vi "FTW-Test-JSON-InvalidPath.vi"() -> (0 "Test Result":errorcluster {"code" format="%.0x"})   [LabVIEW 2015]
uses:
  src/json/FTW-JSON-Type.ctl
  src/json/core/FTW-JSON-Core-Type.ctl
  lib/FTW-KernelFilepath.vi
  src/json/core/FTW-JSON-Core-LibraryReturnValue.vi
  src/error/FTW-ERR-ThrowInvalidReferenceError.vi
  src/json/core/FTW-JSON-Core-ElementType.vi
  codegen/xnode/FTW-JSON-Fetch.xnode
  src/core/type/FTW-Type-JSON.ctl
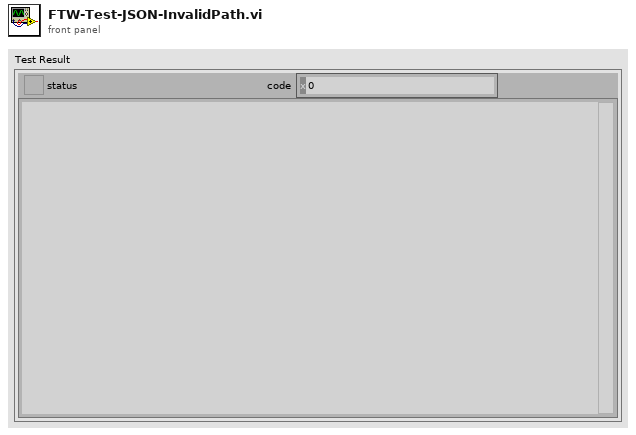
[diagram p1: front panel]
types:
  T1 = typedef "FTW-JSON-Type.ctl" = enum8{"Not Found", "Object", "Array", "String", "Number", "Boolean", "null"}
  T2 = cluster{"Path":string, "ExpectedValue":i32, "ExpectedType":T1, "ExpectedError":bool}[]
  T3 = typedef "FTW-Type-JSON.ctl" = refnum<data-value>
  T4 = typedef "FTW-JSON-Core-Type.ctl" = enum8{"Object", "Array", "String", "Integer", "Floating Point", "true", "false", "null", "undefined"}
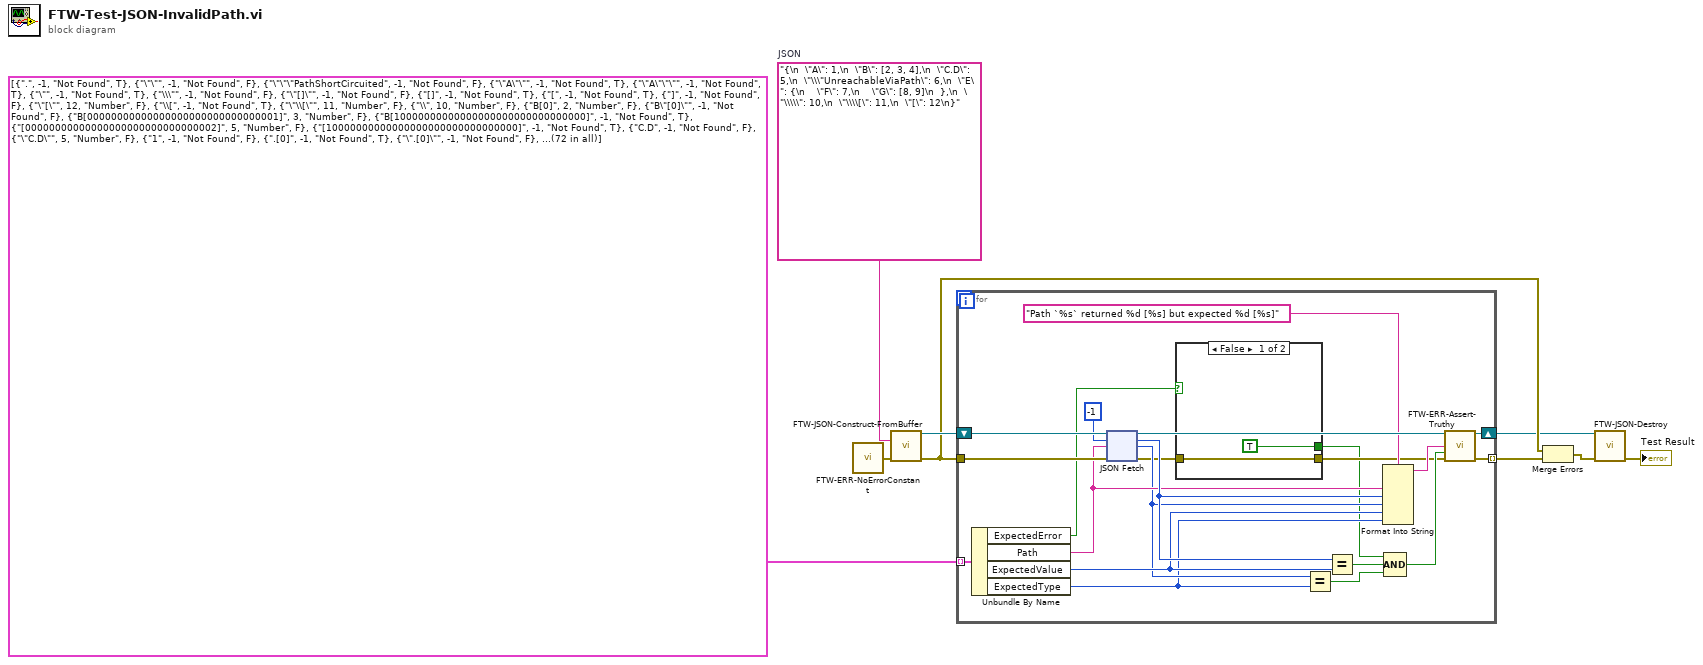
[diagram p0: block diagram]
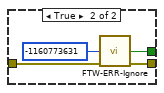
[diagram p2: hidden frame]
diagram:
  w8 = "{\n  \"A\": 1,\n  \"B\": [2, 3, 4],\n  \"C.D\": 5,\n  \"\\\"UnreachableViaPath\": 6,\n  \"E\": {\n    \"F\": 7,\n    \"G\": [8, 9]\n  },\n  \"\\\\\": 10,\n  \"\\\\[\": 11,\n  \"[\": 12\n}"  # JSON
  n1 = call "FTW-ERR-NoErrorConstant.vi"() -> ("no error"=w9:errorcluster)
  n2 = call "FTW-JSON-Construct-FromBuffer.vi"("JSON String (UTF-8)"=w8, "error in"=w9) -> ("JSON"=w7:T3, "error out"=w6:errorcluster)  [unwired: 12 in]
  n3 = for {
    tunnel: w6 -> [w29]
    tunnel: T2 [{"Path"=".", "ExpectedValue"=-1, "ExpectedType"=enum."Not Found", "ExpectedError"=TRUE}, {"Path"="\"\"", "ExpectedValue"=-1, "ExpectedType"=enum."Not Found", "ExpectedError"=FALSE}, {"Path"="\"\"\"PathShortCircuited", "ExpectedValue"=-1, "ExpectedType"=enum."Not Found", "ExpectedError"=FALSE}, {"Path"="\"A\"\"", "ExpectedValue"=-1, "ExpectedType"=enum."Not Found", "ExpectedError"=TRUE}, {"Path"="\"A\"\"\"", "ExpectedValue"=-1, "ExpectedType"=enum."Not Found", "ExpectedError"=TRUE}, {"Path"="\"", "ExpectedValue"=-1, "ExpectedType"=enum."Not Found", "ExpectedError"=TRUE}, {"Path"="\\\"", "ExpectedValue"=-1, "ExpectedType"=enum."Not Found", "ExpectedError"=FALSE}, {"Path"="\"[]\"", "ExpectedValue"=-1, "ExpectedType"=enum."Not Found", "ExpectedError"=FALSE}, {"Path"="[]", "ExpectedValue"=-1, "ExpectedType"=enum."Not Found", "ExpectedError"=TRUE}, {"Path"="[", "ExpectedValue"=-1, "ExpectedType"=enum."Not Found", "ExpectedError"=TRUE}, {"Path"="]", "ExpectedValue"=-1, "ExpectedType"=enum."Not Found", "ExpectedError"=FALSE}, {"Path"="\"[\"", "ExpectedValue"=12, "ExpectedType"=enum."Number", "ExpectedError"=FALSE}, {"Path"="\\[", "ExpectedValue"=-1, "ExpectedType"=enum."Not Found", "ExpectedError"=TRUE}, {"Path"="\"\\[\"", "ExpectedValue"=11, "ExpectedType"=enum."Number", "ExpectedError"=FALSE}, {"Path"="\\", "ExpectedValue"=10, "ExpectedType"=enum."Number", "ExpectedError"=FALSE}, {"Path"="B[0]", "ExpectedValue"=2, "ExpectedType"=enum."Number", "ExpectedError"=FALSE}, {"Path"="B\"[0]\"", "ExpectedValue"=-1, "ExpectedType"=enum."Not Found", "ExpectedError"=FALSE}, {"Path"="B[00000000000000000000000000000001]", "ExpectedValue"=3, "ExpectedType"=enum."Number", "ExpectedError"=FALSE}, {"Path"="B[10000000000000000000000000000000]", "ExpectedValue"=-1, "ExpectedType"=enum."Not Found", "ExpectedError"=TRUE}, {"Path"="[00000000000000000000000000000002]", "ExpectedValue"=5, "ExpectedType"=enum."Number", "ExpectedError"=FALSE}, {"Path"="[10000000000000000000000000000000]", "ExpectedValue"=-1, "ExpectedType"=enum."Not Found", "ExpectedError"=TRUE}, {"Path"="C.D", "ExpectedValue"=-1, "ExpectedType"=enum."Not Found", "ExpectedError"=FALSE}, {"Path"="\"C.D\"", "ExpectedValue"=5, "ExpectedType"=enum."Number", "ExpectedError"=FALSE}, {"Path"="1", "ExpectedValue"=-1, "ExpectedType"=enum."Not Found", "ExpectedError"=FALSE}, {"Path"=".[0]", "ExpectedValue"=-1, "ExpectedType"=enum."Not Found", "ExpectedError"=TRUE}, {"Path"="\".[0]\"", "ExpectedValue"=-1, "ExpectedType"=enum."Not Found", "ExpectedError"=FALSE}, {"Path"="B.2", "ExpectedValue"=-1, "ExpectedType"=enum."Not Found", "ExpectedError"=FALSE}, {"Path"="B.[2]", "ExpectedValue"=-1, "ExpectedType"=enum."Not Found", "ExpectedError"=TRUE}, {"Path"="B.\"[2]\"", "ExpectedValue"=-1, "ExpectedType"=enum."Not Found", "ExpectedError"=FALSE}, {"Path"="[A]", "ExpectedValue"=-1, "ExpectedType"=enum."Not Found", "ExpectedError"=TRUE}, {"Path"="a", "ExpectedValue"=-1, "ExpectedType"=enum."Not Found", "ExpectedError"=FALSE}, {"Path"="][", "ExpectedValue"=-1, "ExpectedType"=enum."Not Found", "ExpectedError"=FALSE}, {"Path"="\"UnreachableViaPath", "ExpectedValue"=-1, "ExpectedType"=enum."Not Found", "ExpectedError"=TRUE}, {"Path"="\"\"UnreachableViaPath\"PathShortCircuited", "ExpectedValue"=-1, "ExpectedType"=enum."Not Found", "ExpectedError"=FALSE}, {"Path"="\\\"UnreachableViaPath", "ExpectedValue"=-1, "ExpectedType"=enum."Not Found", "ExpectedError"=FALSE}, {"Path"="[3]", "ExpectedValue"=6, "ExpectedType"=enum."Number", "ExpectedError"=FALSE}, {"Path"="E.F", "ExpectedValue"=7, "ExpectedType"=enum."Number", "ExpectedError"=FALSE}, {"Path"="\"E.F\"", "ExpectedValue"=-1, "ExpectedType"=enum."Not Found", "ExpectedError"=FALSE}, {"Path"="E.F\"", "ExpectedValue"=-1, "ExpectedType"=enum."Not Found", "ExpectedError"=FALSE}, {"Path"="\"E.F", "ExpectedValue"=-1, "ExpectedType"=enum."Not Found", "ExpectedError"=TRUE}, {"Path"="E[]", "ExpectedValue"=-1, "ExpectedType"=enum."Not Found", "ExpectedError"=TRUE}, {"Path"="E[-1]", "ExpectedValue"=-1, "ExpectedType"=enum."Not Found", "ExpectedError"=TRUE}, {"Path"="E[0]", "ExpectedValue"=7, "ExpectedType"=enum."Number", "ExpectedError"=FALSE}, {"Path"="E[F]", "ExpectedValue"=-1, "ExpectedType"=enum."Not Found", "ExpectedError"=TRUE}, {"Path"="[E][F]", "ExpectedValue"=-1, "ExpectedType"=enum."Not Found", "ExpectedError"=TRUE}, {"Path"="[E]", "ExpectedValue"=-1, "ExpectedType"=enum."Not Found", "ExpectedError"=TRUE}, {"Path"="[\"E\"]", "ExpectedValue"=-1, "ExpectedType"=enum."Not Found", "ExpectedError"=TRUE}, {"Path"="\"[E]\"", "ExpectedValue"=-1, "ExpectedType"=enum."Not Found", "ExpectedError"=FALSE}, {"Path"="[4]F", "ExpectedValue"=-1, "ExpectedType"=enum."Not Found", "ExpectedError"=TRUE}, {"Path"="[4].F", "ExpectedValue"=7, "ExpectedType"=enum."Number", "ExpectedError"=FALSE}, {"Path"="[4].[0]", "ExpectedValue"=-1, "ExpectedType"=enum."Not Found", "ExpectedError"=TRUE}, {"Path"="[4][0]", "ExpectedValue"=7, "ExpectedType"=enum."Number", "ExpectedError"=FALSE}, {"Path"="[4][1][0]", "ExpectedValue"=8, "ExpectedType"=enum."Number", "ExpectedError"=FALSE}, {"Path"="[4].G", "ExpectedValue"=-1, "ExpectedType"=enum."Array", "ExpectedError"=FALSE}, {"Path"="E.G.[0]", "ExpectedValue"=-1, "ExpectedType"=enum."Not Found", "ExpectedError"=TRUE}, {"Path"="E.G[0]", "ExpectedValue"=8, "ExpectedType"=enum."Number", "ExpectedError"=FALSE}, {"Path"="E.G[]", "ExpectedValue"=-1, "ExpectedType"=enum."Not Found", "ExpectedError"=TRUE}, {"Path"="[E.G[0]]", "ExpectedValue"=-1, "ExpectedType"=enum."Not Found", "ExpectedError"=TRUE}, {"Path"="\"E.G[0]\"", "ExpectedValue"=-1, "ExpectedType"=enum."Not Found", "ExpectedError"=FALSE}, {"Path"="[00000004][00000001][00000000]", "ExpectedValue"=8, "ExpectedType"=enum."Number", "ExpectedError"=FALSE}, {"Path"="..", "ExpectedValue"=-1, "ExpectedType"=enum."Not Found", "ExpectedError"=TRUE}, {"Path"=".\".\"", "ExpectedValue"=-1, "ExpectedType"=enum."Not Found", "ExpectedError"=FALSE}, {"Path"=".[0]", "ExpectedValue"=-1, "ExpectedType"=enum."Not Found", "ExpectedError"=TRUE}, {"Path"=".\"[0]\"", "ExpectedValue"=-1, "ExpectedType"=enum."Not Found", "ExpectedError"=FALSE}, {"Path"=".A", "ExpectedValue"=1, "ExpectedType"=enum."Number", "ExpectedError"=FALSE}, {"Path"=".\"A\"", "ExpectedValue"=1, "ExpectedType"=enum."Number", "ExpectedError"=FALSE}, {"Path"=".A.", "ExpectedValue"=-1, "ExpectedType"=enum."Not Found", "ExpectedError"=TRUE}, {"Path"=".E.F", "ExpectedValue"=7, "ExpectedType"=enum."Number", "ExpectedError"=FALSE}, {"Path"=".E[0]", "ExpectedValue"=7, "ExpectedType"=enum."Number", "ExpectedError"=FALSE}, {"Path"=" ", "ExpectedValue"=-1, "ExpectedType"=enum."Not Found", "ExpectedError"=FALSE}, {"Path"="", "ExpectedValue"=-1, "ExpectedType"=enum."Object", "ExpectedError"=FALSE}, {"Path"=".", "ExpectedValue"=-1, "ExpectedType"=enum."Not Found", "ExpectedError"=TRUE}] -> [w28] mode=indexing
    shift-right: [w27] -> w2
    shift-left: w7 -> [w21]
    tunnel: [w25] -> w5 mode=indexing
    n4 = Unbundle By Name(w28) -> ("ExpectedError"=w14:bool, "Path"=w20:string, "ExpectedValue"=w22:i32, "ExpectedType"=w15:T1)
    n5 = xnode "JSON Fetch"("JSON"=w21, "Element Type and Default Value"=-1, "Element Path"=w20, "error in"=w29) -> ("JSON out"=w27:T3, "Value"=w23:i32, "JSON Element Type"=w16:T1, "error out"=w13:errorcluster)  [unwired: 1 in]
    n6 = case shown="False" w14 {
      tunnel: w13 -> [w31 w34]
      tunnel: [w31 w33] -> w12
      tunnel: [TRUE ("Error Cleared?") w32] -> w11
      frame False {
      }
      frame True {
        n7 = call "FTW-ERR-Ignore.vi"("Error Code"=-1160773631, "error in"=w34) -> ("Error Cleared?"=w32:bool, "error out"=w33:errorcluster)  [unwired: 12 in]
      }
    }
    n8 = Equal?(x=w16, y=w15) -> (x = y?=w18:bool)
    n9 = Equal?(x=w23, y=w22) -> (x = y?=w19:bool)
    n10 = Format Into String(format string="Path `%s` returned %d [%s] but expected %d [%s]" ("Assertion"), w20, w23, w16, w22, w15) -> (resulting string=w24:string)  [unwired: 2 in, 1 out]
    n11 = Compound Arithmetic op=AND(w11, w19, w18) -> (w17:bool)
    n12 = call "FTW-ERR-Assert-Truthy.vi"("Assertion"=w24, "Assertion holds true?"=w17, "error in"=w12) -> ("error out"=w25:errorcluster)  [unwired: 12 in]
  }
  n13 = Merge Errors(w6, w5) -> (w1:errorcluster)
  n14 = call "FTW-JSON-Destroy.vi"("JSON"=w2, "error in"=w1) -> ("error out"=→"Test Result":errorcluster)  [unwired: 13 in]
